vi "Table Set Value To All.vi"(4 "Column Size":i32=-1, 6 "Row Size":i32=-1, 8 "error in":errorcluster, 9 "String":string, 11 "Table Ref In":refnum<vi>) -> (0 "error out":errorcluster, 3 "Table Ref Out":refnum<vi>)   [LabVIEW 2024]
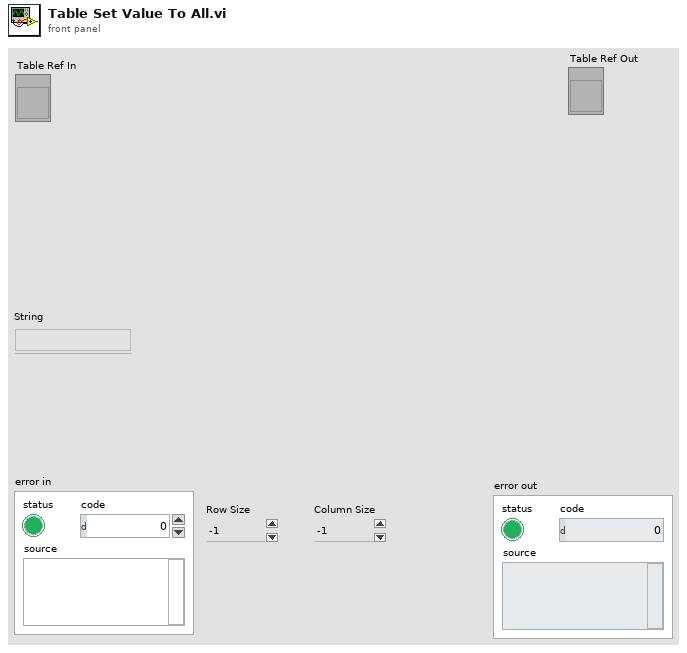
[diagram p1: front panel]
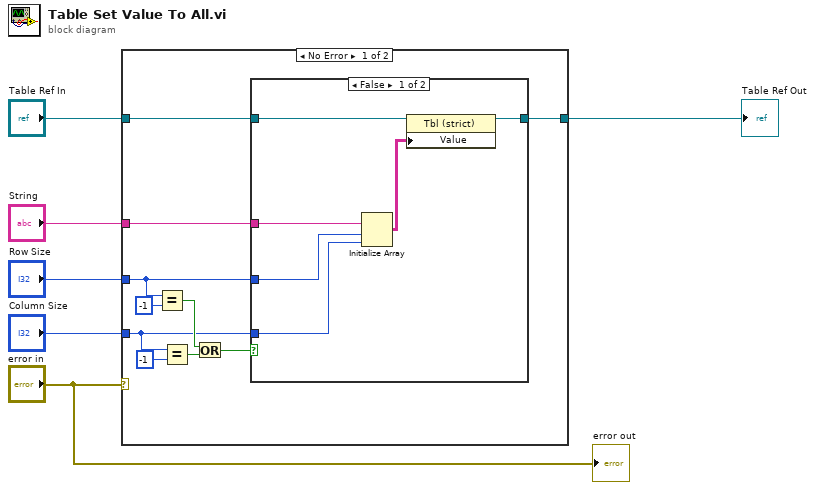
[diagram p0: block diagram]
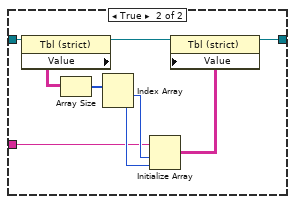
[diagram p2: hidden frame]
diagram:
  n1 = case shown="No Error" "error in" {
    tunnel: "Table Ref In" -> [w16 w32]
    tunnel: [w15 w32] -> w5
    tunnel: "String" -> [w14 _]
    tunnel: "Row Size" -> [w8 _]
    tunnel: "Column Size" -> [w7 _]
    frame No Error {
      n2 = Equal?(x=w8, y=-1) -> (x = y?=w10:bool)
      n3 = Equal?(x=w7, y=-1) -> (x = y?=w11:bool)
      n4 = Or(x=w10, y=w11) -> (x .or. y?=w9:bool)
      n5 = case shown="False" w9 {
        tunnel: w16 -> [w22 w25]
        tunnel: [w21 w24] -> w15
        tunnel: w14 -> [w20 w23]
        tunnel: w8 -> [w18 _]
        tunnel: w7 -> [w17 _]
        frame False {
          n6 = Initialize Array(w20, w18, w17) -> (w19:string[][])
          n7 = property class="Tbl (strict)"(reference=w22, "Value"=w19) -> (reference out=w21:refnum<vi>)  [unwired: 1 in, 1 out]
        }
        frame True {
          n8 = property class="Tbl (strict)"(reference=w25) -> (reference out=w31:refnum<vi>, "Value"=w30:string[][])  [unwired: 1 in, 1 out]
          n9 = Array Size(array=w30) -> (size(s)=w29:i32[])
          n10 = Index Array(array=w29) -> (element #1=w28:i32, element #2=w27:i32)  [unwired: 2 in]
          n11 = Initialize Array(w23, w28, w27) -> (w26:string[][])
          n12 = property class="Tbl (strict)"(reference=w31, "Value"=w26) -> (reference out=w24:refnum<vi>)  [unwired: 1 in, 1 out]
        }
      }
    }
    frame Error {
    }
  }
  "Table Ref Out" <- w5
  "error out" <- "error in"
